vi "Add Customer.vi"(7 "Time scale [ms]":u32=5000, 8 "error in (no error)":errorcluster, 10 "Name":string, 11 "Coffee Shop in":refnum<class "Coffee Shop.lvclass">) -> (0 "error out":errorcluster, 3 "Coffee Shop out":refnum<class "Coffee Shop.lvclass">)   [LabVIEW 2020, in "Coffee Shop.lvclass"]
uses:
  Coffee Shop.lvclass
  C:/Program Files (x86)/National Instruments/LabVIEW 2020/vi.lib/Astemes/Triarc Framework/Process/Process.lvclass
  People/Customers/Customer/Customer.lvclass
  C:/git/astemes-triarc-examples/source/Coffee Shop/Processes/People/Person/Person.lvclass
  <vilib>/Astemes/Triarc Framework/Process/Process.lvclass/Process.ctl
  People/Person/Person.lvclass/Person.ctl
  <vilib>/Astemes/Triarc Framework/Process/Private/SubVIs/Handle Debug Data.vi
  <vilib>/Astemes/Triarc Framework/Logging/Log Debug.vi
  <vilib>/AdvancedString/1D String Array to Delimited String.vi
  <vilib>/Utility/High Resolution Relative Seconds.vi
  People/Person/Person.lvclass
  <vilib>/Astemes/Triarc Framework/Process/Public/Lifecycle/Get Lifecycle State.vi
  <vilib>/Astemes/Triarc Framework/Process/Public/Read Name.vi
  <vilib>/Astemes/Triarc Framework/Callback/Callback.lvclass
  <vilib>/Astemes/Triarc Framework/Process/Process.lvclass
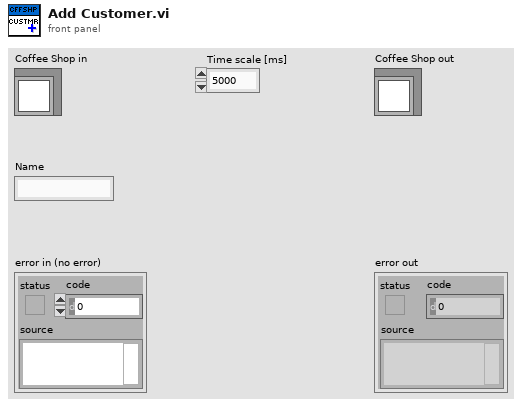
[diagram p1: front panel]
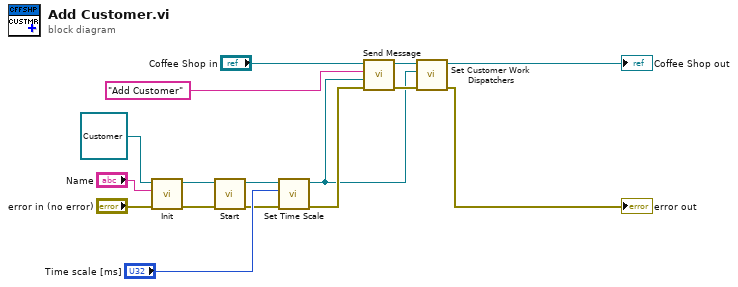
[diagram p0: block diagram]
diagram:
  n1 = call-dynamic "Init.vi"("error in (no error)"="error in (no error)", "Name"="Name", "View In"=refnum<class "Customer.lvclass"> refnum ("Customer.lvclass")) -> ("error out"=w10:errorcluster, "View Out"=w2:refnum<class "Customer.lvclass">)  [unwired: 7 in]
  n2 = call <vilib>:"Start.vi"("error in (no error)"=w10, "Process In"=w2) -> ("error out"=w3:errorcluster, "Process Out"=w1:refnum<class "Customer.lvclass">)  [unwired: 7 in, 1 out]
  n3 = call "Set Time Scale.vi"("TRIARC_ERROR_IN"=w3, "Time Scale [ms]"="Time scale [ms]", "Person In"=w1) -> ("TRIARC_ERROR_OUT"=w6:errorcluster, "Person Out"=w5:refnum<class "Customer.lvclass">)  [unwired: 7 in]
  n4 = call <vilib>:"Send Message.vi"("error in (no error)"=w6, "Message Data"=w5, "Message"="Add Customer", "Process In"="Coffee Shop in") -> ("error out"=w16:errorcluster, "Process Out"=w9:refnum<class "Coffee Shop.lvclass">)  [unwired: 6 in]
  n5 = call "Set Customer Work Dispatchers.vi"("error in (no error)"=w16, "Customer"=w5, "Coffee Shop In"=w9) -> ("error out"=→"error out":errorcluster, "Coffee Shop Out"=→"Coffee Shop out":refnum<class "Coffee Shop.lvclass">)  [unwired: 7 in]
